vi "VDA Scan Device.vi"(8 "error in (no error)":errorcluster, 11 "NeedInit":u8) -> (0 "error out":errorcluster, 3 "function return":i32)   [LabVIEW 2010, in "CntrolDAC.lvlib"]
doc: "int WINAPI VDA_ScanDevice(unsigned char NeedInit=1);"
uses:
  CntrolDAC.lvlib
  labview_32bit/ControlDAC/Ginkgo_Driver.dll
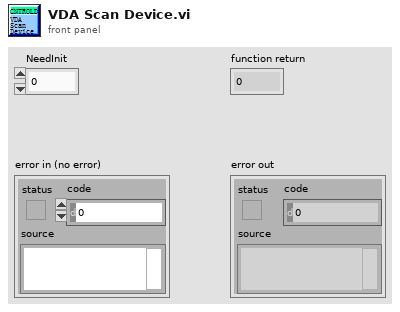
[diagram p1: front panel]
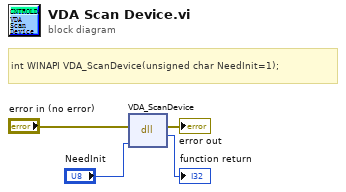
[diagram p0: block diagram]
diagram:
  # "int WINAPI VDA_ScanDevice(unsigned char NeedInit=1);"
  n1 = dll-call lib="E:/Project/vt_ginkgo/truck/Ginkgo Driver/vs2010/Ginkgo_USB-I2C&SPI&CAN_API_v2.0.3.3/lib/labview_32bit/ControlDAC/Ginkgo_Driver.*" fn="VDA_ScanDevice"(error in="error in (no error)", "NeedInit"="NeedInit") -> (error out=→"error out":errorcluster, →"function return":i32)  [unwired: 3 in, 1 out]
